vi "createScanPoints.vi"(8 "travelRange":cluster{"X":dbl, "Y":dbl, "Z":dbl}, 9 "pBot_scanN":cluster{"X":u16, "Y":u16, "Z":u16}, 10 "pBot_minScanRegion":cluster{"X":sgl, "Y":sgl, "Z":sgl}, 11 "pBot_maxScanRegion":cluster{"X":sgl, "Y":sgl, "Z":sgl}) -> (3 "scanPoints":T1)   [LabVIEW 2015]
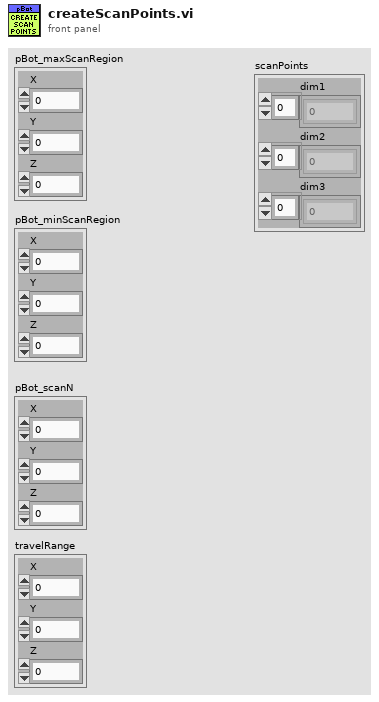
[diagram p1: front panel]
types:
  T1 = cluster{"dim1":sgl[], "dim2":sgl[], "dim3":sgl[]}
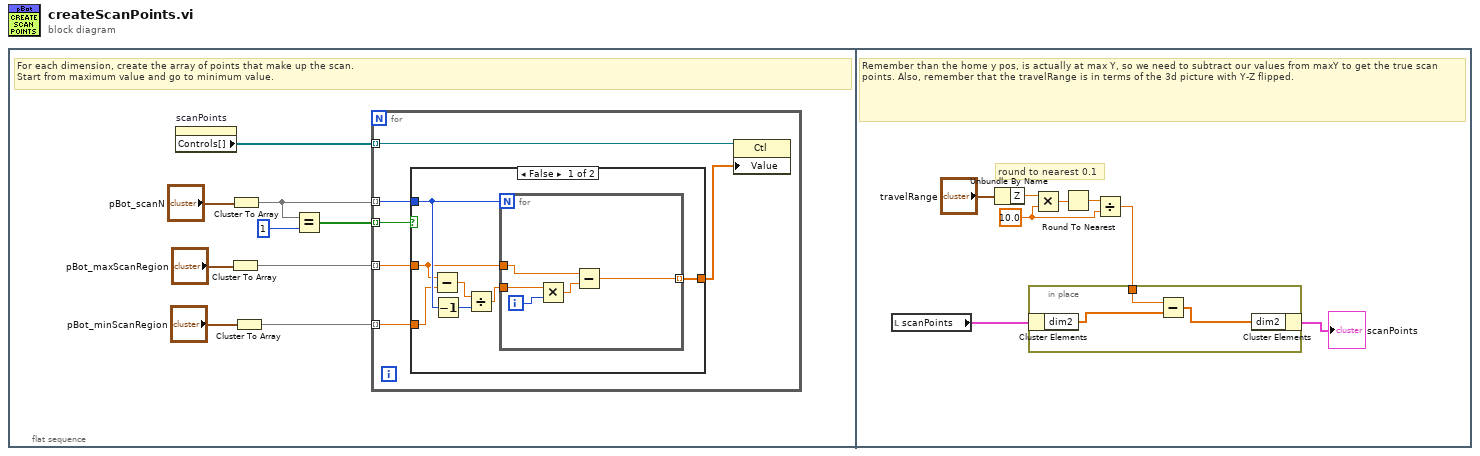
[diagram p0: block diagram]
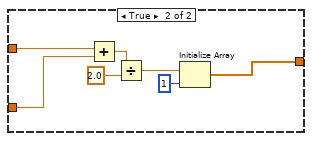
[diagram p2: hidden frame]
diagram:
  n1 = flat-sequence {
    frame #0 {
      # "For each dimension, create the array of points that make up the scan.\nStart from maximum value and go to minimum value."
      n2 = property on="scanPoints" class="Clust (strict)"() -> ("Controls[]"=w1:refnum<vi>[])  [unwired: 2 in, 2 out]
      n3 = Cluster To Array(cluster="pBot_maxScanRegion") -> (array=w5:sgl[])
      n4 = Cluster To Array(cluster="pBot_scanN") -> (array=w4:u16[])
      n5 = Cluster To Array(cluster="pBot_minScanRegion") -> (array=w6:sgl[])
      n6 = Equal?(x=w4, y=u16 1 ("X")) -> (x = y?=w2:bool[])
      n7 = for {
        tunnel: w2 -> [w15] mode=indexing
        tunnel: w4 -> [w12] mode=indexing
        tunnel: w6 -> [w13] mode=indexing
        tunnel: w5 -> [w14] mode=indexing
        tunnel: w1 -> [w11] mode=indexing
        n8 = case shown="False" w15 {
          tunnel: w14 -> [w16 w34]
          tunnel: w13 -> [w18 w33]
          tunnel: [w17 w28] -> w10
          tunnel: w12 -> [w20 _]
          frame False {
            n9 = Subtract(x=w16, y=w18) -> (x-y=w22:sgl)
            n10 = Decrement(x=w20) -> (x-1=w21:u16)
            n11 = Divide(x=w22, y=w21) -> (x/y=w19:sgl)
            n12 = for {
              N: w20 -> [_]
              tunnel: w19 -> [w27]
              tunnel: [w25] -> w17 mode=indexing
              tunnel: w16 -> [w24]
              i -> [w26]
              n13 = Multiply(x=w27, y=w26) -> (x*y=w23:sgl)
              n14 = Subtract(x=w24, y=w23) -> (x-y=w25:sgl)
            }
          }
          frame True {
            n15 = Add(x=w34, y=w33) -> (x+y=w32:sgl)
            n16 = Divide(x=w32, y=sgl 2.0) -> (x/y=w30:sgl)
            n17 = Initialize Array(w30, 1 ("dimension size")) -> (w28:sgl[])
          }
        }
        n18 = property class="Ctl"(reference=w11, "Value"=w10) -> ()  [unwired: 1 in, 2 out]
      }
    }
    frame #1 {
      w38 = 10.0
      # "round to nearest 0.1"
      # "Remember than the home y pos, is actually at max Y, so we need to subtract our values from maxY to get the true scan points. Also, remember that the travelRange is in terms of the 3d picture with Y-Z flipped."
      n19 = local read "scanPoints"() -> (w37:T1)
      n20 = Unbundle By Name("travelRange") -> ("Z"=w41:dbl)
      n21 = Multiply(x=w41, y=w38) -> (x*y=w40:dbl)
      n22 = Round To Nearest(number=w40) -> (nearest integer value=w39:dbl)
      n23 = Divide(x=w39, y=w38) -> (x/y=w36:dbl)
      n24 = in-place {
        in-place-border: w36 -> [w45]
        n25 = in-place-cluster #1(w37) -> ("dim2"=w44:sgl[])
        n26 = Subtract(x=w45, y=w44) -> (x-y=w43:dbl[])
        n27 = in-place-cluster #1("dim2"=w43) -> (→"scanPoints":T1)
      }
    }
  }
